vi "Find Actor Core.vi"() -> (2 "Actor Cores":string[](array[string]))   [LabVIEW 2017, in "MGI-Monitored Actor Core.lvlib" / "Monitored Actor.lvclass"]
doc: "Looks through the call chain to find the correct version of actor core. We the Child's specific implementation of actor core if possible.\n\nBecause this will look through the call chain, this VI only works if it's run in a do method of an actor. (Not in pre-launch init for example)\n----\nCopyright: MGI 2018\nAuthor: Derek Trepanier"
uses:
  Monitored Actor.lvclass
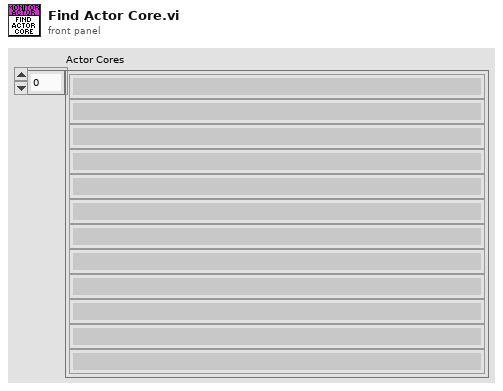
[diagram p1: front panel]
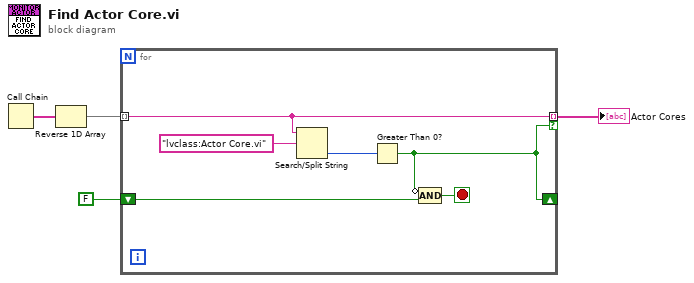
[diagram p0: block diagram]
diagram:
  n1 = Call Chain() -> (call chain=w3:string[])
  n2 = Reverse 1D Array(array=w3) -> (reversed array=w2:string[])
  n3 = for {
    tunnel: w2 -> [w7] mode=indexing
    tunnel: [w7] -> w4 mode=indexing if=w8
    shift-right: [w8] -> _
    shift-left: FALSE -> [w10]
    stop <- w9 stop-if-true
    n4 = Search/Split String(string=w7, search string/char (-)="lvclass:Actor Core.vi" ("search string")) -> (offset of match=w5:i32)  [unwired: 1 in, 2 out]
    n5 = Greater Than 0?(x=w5) -> (x > 0?=w8:bool)
    n6 = Compound Arithmetic op=AND(invert w8, w10) -> (w9:bool)
  }
  "Actor Cores" <- w4
